vi "Motor Controller Datastream (get N samples).vi"(8 "N samples":i32, 9 "Set data rate?":bool, 10 "Data rate (Hz)":u8(ring)=14 items=["1", "2", "4", "5", "8", "10", "16", "20", "25", "32", "40", "50", "64", "80", "100", "125", "160", "200", "250", "320", "400", "500", "625", "800", "1000"], 11 "COM port":refnum<visa-resource-name>) -> (0 "Error out":errorcluster, 1 "Chk err":u32, 2 "Frm err":u32, 3 "Data cluster array":T1[](array[typedef]))   [LabVIEW 2020]
uses:
  ctls/CTRL_Data_Out.ctl
  ctls/CTRL_Cmd.ctl
panel:
  in  "Stop":bool
  out "Datastream":T2(graph)
  # "RPM (/min)"
  # "I_m (A)"
  # "Photo (V)"
  # "Duty ()"
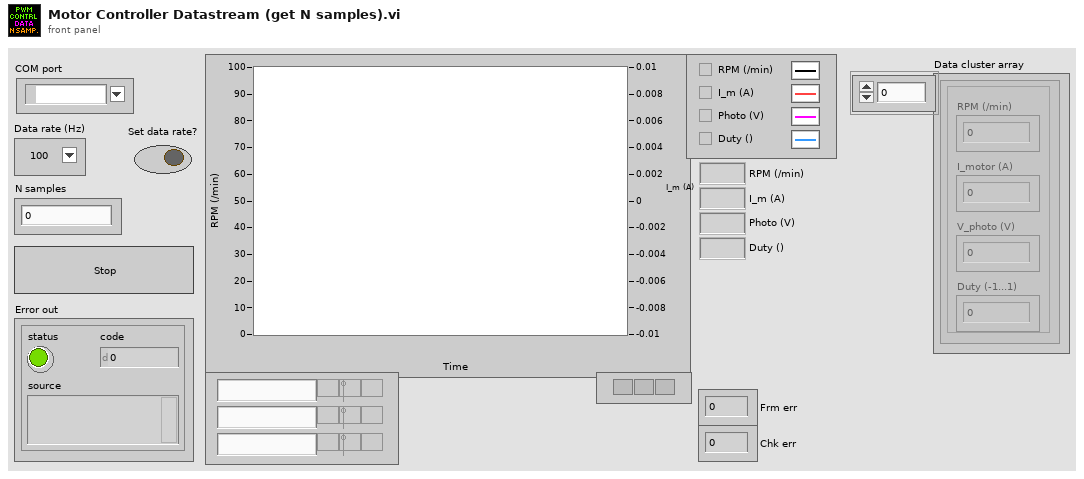
[diagram p1: front panel]
types:
  T1 = typedef "CTRL_Data_Out.ctl" = cluster{"RPM (/min)":sgl, "I_motor (A)":sgl, "V_photo (V)":sgl, "Duty (-1...1)":sgl}
  T2 = cluster{"RPM (/min)":sgl, "I_motor (A)":sgl, "V_photo (V)":sgl, "Duty (-1...1)":sgl}
  T3 = cluster{"RPM (/min)":sgl, "I_motor (A)":sgl, "V_photo (V)":sgl, "Duty (-1...1)":sgl}[]
  T4 = typedef "CTRL_Cmd.ctl" = string
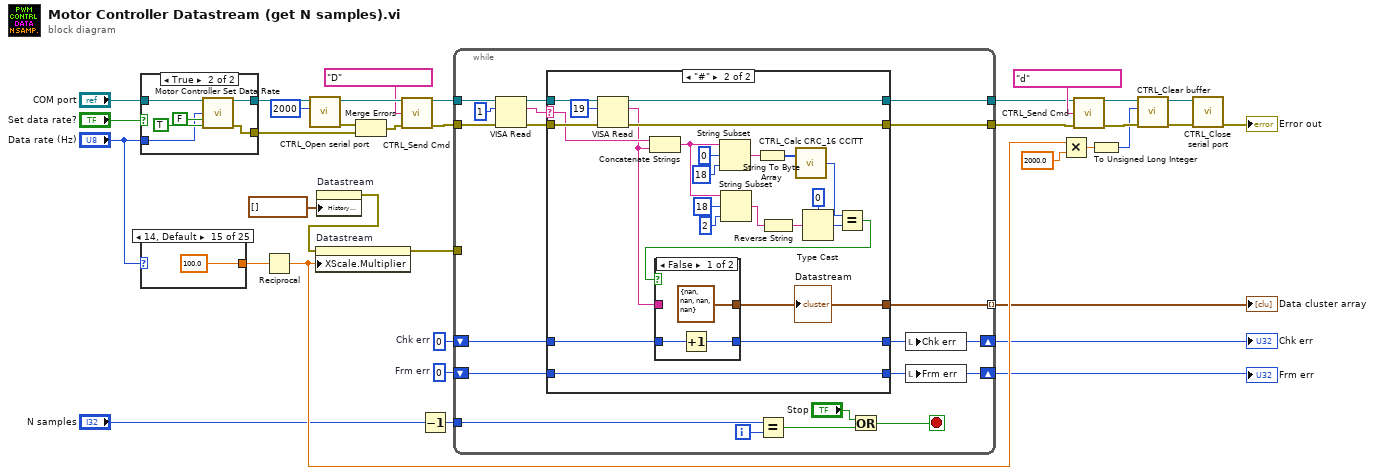
[diagram p0: block diagram]
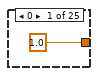
[diagram p2: hidden frame]
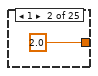
[diagram p3: hidden frame]
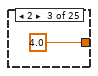
[diagram p4: hidden frame]
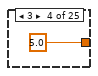
[diagram p5: hidden frame]
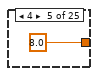
[diagram p6: hidden frame]
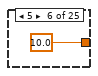
[diagram p7: hidden frame]
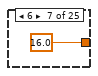
[diagram p8: hidden frame]
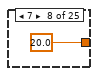
[diagram p9: hidden frame]
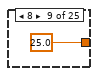
[diagram p10: hidden frame]
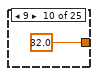
[diagram p11: hidden frame]
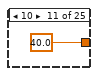
[diagram p12: hidden frame]
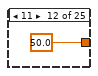
[diagram p13: hidden frame]
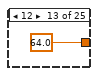
[diagram p14: hidden frame]
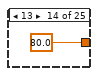
[diagram p15: hidden frame]
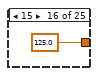
[diagram p16: hidden frame]
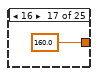
[diagram p17: hidden frame]
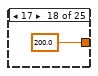
[diagram p18: hidden frame]
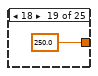
[diagram p19: hidden frame]
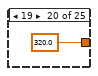
[diagram p20: hidden frame]
diagram:
  w9 = u32 0  # Chk err
  w10 = u32 0  # Frm err
  n1 = case shown="True" "Set data rate?" {
    tunnel: "COM port" -> [w37 w43]
    tunnel: [w37 w42] -> w15
    tunnel: [errorcluster {"status"=FALSE, "code"=0, "source"=""} ("Error out") w41] -> w12
    tunnel: "Data rate (Hz)" -> [_ w38]
    frame False {
    }
    frame True {
      n2 = call "Motor Controller Set Data Rate.vi"("COM port"=w43, "Data rate (Hz)"=w38, "Set as power-on default"=FALSE, "Close port after action"=TRUE) -> ("COM port out"=w42:refnum<visa-resource-name>, "Error out"=w41:errorcluster)  [unwired: 10 in]
    }
  }
  n3 = case shown="14, Default" "Data rate (Hz)" {
    tunnel: [1.0 2.0 4.0 5.0 8.0 10.0 16.0 20.0 25.0 32.0 40.0 50.0 64.0 80.0 100.0 125.0 160.0 200.0 250.0 320.0 400.0 500.0 625.0 800.0 1000.0] -> w2
    frame 0 {
    }
    frame 1 {
    }
    frame 2 {
    }
    frame 3 {
    }
    frame 4 {
    }
    frame 5 {
    }
    frame 6 {
    }
    frame 7 {
    }
    frame 8 {
    }
    frame 9 {
    }
    frame 10 {
    }
    frame 11 {
    }
    frame 12 {
    }
    frame 13 {
    }
    frame 14, Default {
    }
    frame 15 {
    }
    frame 16 {
    }
    frame 17 {
    }
    frame 18 {
    }
    frame 19 {
    }
    frame 20 {
    }
    frame 21 {
    }
    frame 22 {
    }
    frame 23 {
    }
    frame 24 {
    }
  }
  n4 = Reciprocal(x=w2) -> (1/x=w11:dbl)
  n5 = call "CTRL_Open serial port.vi"("timeout (ms)"=u32 2000, "VISA resource name"=w15) -> ("Error out"=w14:errorcluster, "VISA resource name out"=w19:refnum<visa-resource-name>)  [unwired: 8 in]
  n6 = property on="Datastream" class="WFChart (strict)"("History Data"=T3 []) -> (error out=w31:errorcluster)  [unwired: 2 in, 1 out]
  n7 = property on="Datastream" class="WFChart (strict)"(error in=w31, "XScale.Multiplier"=w11) -> (error out=w22:errorcluster)  [unwired: 1 in, 1 out]
  n8 = Merge Errors(w14, w12) -> (w13:errorcluster)
  n9 = call "CTRL_Send Cmd.vi"("Port"=w19, "Cmd"=T4 "D" ("Command"), "Error In"=w13) -> ("Port out"=w20:refnum<visa-resource-name>, "Error Out"=w21:errorcluster)  [unwired: 11 in]
  n10 = Decrement(x="N samples") -> (x-1=w5:i32)
  n11 = while {
    tunnel: w20 -> [w86]
    tunnel: w21 -> [w85]
    tunnel: [w80] -> w28
    tunnel: [w79] -> w29
    tunnel: w22 -> [_]
    shift-right: [w69] -> w3
    shift-left: w10 -> [w78]
    shift-right: [w70] -> w4
    shift-left: w9 -> [w77]
    tunnel: [w76] -> w7 mode=indexing
    tunnel: w5 -> [w75]
    i -> [w73]
    stop <- w74 stop-if-true
    n12 = VISA Read(VISA resource name=w86, byte count=u32 1, error in (no error)=w85) -> (VISA resource name out=w82:refnum<visa-resource-name>, read buffer=w81:string, error out=w83:errorcluster)  [unwired: 1 out]
    n13 = case shown="\"#\"" w81 {
      selector: w81 -> [_ w111]
      tunnel: w83 -> [w92 w115]
      tunnel: w82 -> [w91 w116]
      tunnel: [w92 w113] -> w80
      tunnel: [w91 w112] -> w79
      tunnel: [w90 w96] -> w69
      tunnel: w78 -> [w89 w96]
      tunnel: [w88 w93] -> w70
      tunnel: w77 -> [w88 w95]
      tunnel: [T1 {"RPM (/min)"=nan, "I_motor (A)"=nan, "V_photo (V)"=nan, "Duty (-1...1)"=nan} ("Data") w94] -> w76
      frame Default {
        n14 = Increment(x=w89) -> (x+1=w90:u32)
      }
      frame "#" {
        n15 = VISA Read(VISA resource name=w116, byte count=u32 19, error in (no error)=w115) -> (VISA resource name out=w112:refnum<visa-resource-name>, read buffer=w110:string, error out=w113:errorcluster)  [unwired: 1 out]
        n16 = Concatenate Strings(w111, w110) -> (w98:string)
        n17 = String Subset(string=w98, offset (0)=0, length (rest)=18 ("length (rest)")) -> (substring=w97:string)
        n18 = String Subset(string=w98, offset (0)=18, length (rest)=2 ("length (rest)")) -> (substring=w106:string)
        n19 = String To Byte Array(string=w97) -> (unsigned byte array=w109:u8[])
        n20 = Reverse String(1:w106) -> (0:w104:string)
        n21 = call "CTRL_Calc CRC_16 CCITT.vi"("Data bytes"=w109) -> ("CRC_16-CCITT"=w103:u16)  [unwired: 1 in]
        n22 = Type Cast(type=u16 0 ("length (rest)"), x=w104) -> (*(type *) &x=w102:u16)
        n23 = Equal?(x=w103, y=w102) -> (x = y?=w101:bool)
        n24 = case shown="False" w101 {
          tunnel: w110 -> [_ w122]
          tunnel: [T1 {"RPM (/min)"=nan, "I_motor (A)"=nan, "V_photo (V)"=nan, "Duty (-1...1)"=nan} ("Data") w121] -> w94
          tunnel: [w119 w120] -> w93
          tunnel: w95 -> [w118 w120]
          frame False {
            n25 = Increment(x=w118) -> (x+1=w119:u32)
          }
          frame True {
            n26 = call "CTRL_Convert serial string to Eng vals.vi"("Serial buffer string (excluding FrameChar)"=w122) -> ("Data"=w121:T1)
          }
        }
        "Datastream" <- w94
      }
    }
    n27 = Equal?(x=w75, y=w73) -> (x = y?=w72:bool)
    n28 = Or(x="Stop", y=w72) -> (x .or. y?=w74:bool)
    n29 = local write "Chk err"(w70) -> ()
    n30 = local write "Frm err"(w69) -> ()
  }
  "Data cluster array" <- w7
  "Chk err" <- w4
  "Frm err" <- w3
  n31 = Multiply(x=w11, y=2000.0) -> (x*y=w25:dbl)
  n32 = call "CTRL_Send Cmd.vi"("Port"=w29, "Cmd"=T4 "d" ("Command"), "Error In"=w28) -> ("Port out"=w27:refnum<visa-resource-name>, "Error Out"=w26:errorcluster)  [unwired: 11 in]
  n33 = To Unsigned Long Integer(number=w25) -> (unsigned 32bit integer=w23:u32)
  n34 = call "CTRL_Clear buffer.vi"("Error in"=w26, "dt for timeout (ms)"=w23, "VISA resource name in"=w27) -> ("Error out"=w33:errorcluster, "VISA resource name out"=w34:refnum<visa-resource-name>)  [unwired: 3 in]
  n35 = call "CTRL_Close serial port.vi"("Error in"=w33, "VISA resource name"=w34) -> ("Error out"=→"Error out":errorcluster)  [unwired: 9 in]
